vi "Giao tiep 2.vi"() -> ()   [LabVIEW 2020]
uses:
  <vilib>/Instr/_visa.llb/VISA Configure Serial Port (Instr).vi
panel:
  out "concatenated string":string
  in  "BnhanMT":i32(slide) scale=0.0..255.0
  in  "AnhanMT":i32(slide) scale=0.0..255.0
  out "BguiMT":i32
  out "AguiMT":i32
  out "htB":i32(knob) scale=0.0..1000.0
  out "htA":i32(knob) scale=0.0..1023.0
  in  "VISA resource name":refnum<visa-resource-name>="COM10"
  in  "stop":bool
  # "Toc do: 115200"
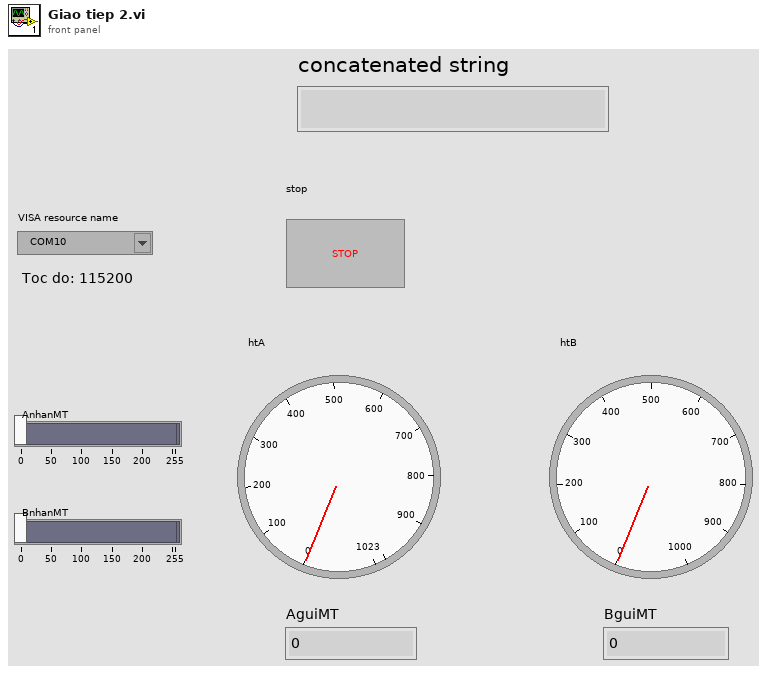
[diagram p1: front panel]
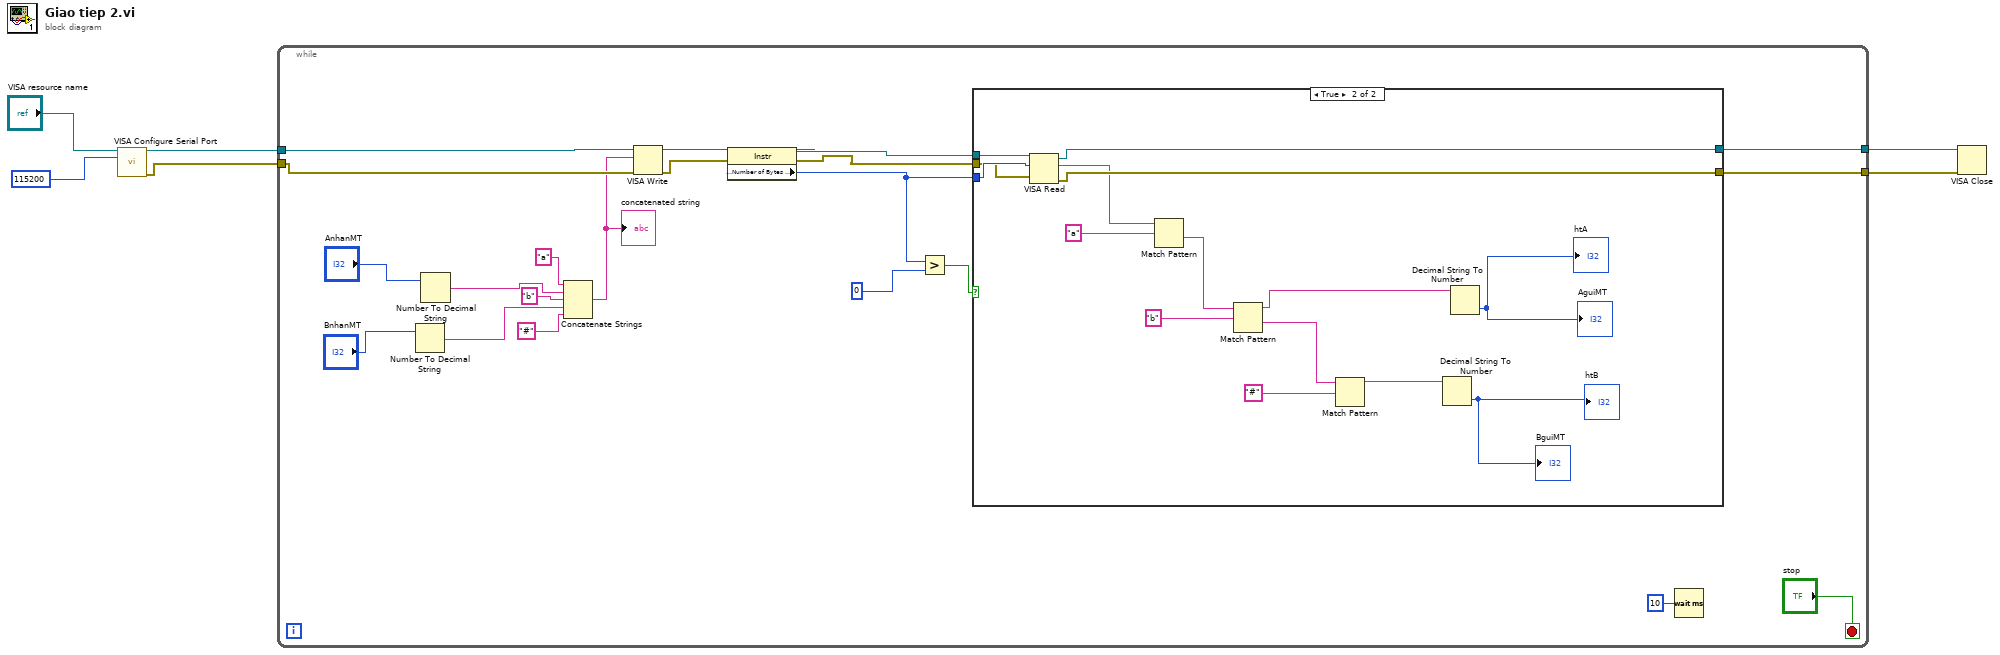
[diagram p0: block diagram]
diagram:
  n1 = call-poly "VISA Configure Serial Port"("VISA resource name"="VISA resource name", "baud rate (9600)"=u32 115200) -> ("VISA resource name out"=w4:refnum<visa-resource-name>, "error out"=w2:errorcluster)  [unwired: 12 in]
  n2 = while {
    tunnel: w4 -> [w21]
    tunnel: [w24] -> w3
    tunnel: w2 -> [w19]
    tunnel: [w22] -> w1
    stop <- "stop" stop-if-true
    n3 = Number To Decimal String(number="BnhanMT") -> (decimal integer string=w9:string)  [unwired: 1 in]
    n4 = Number To Decimal String(number="AnhanMT") -> (decimal integer string=w11:string)  [unwired: 1 in]
    n5 = Concatenate Strings("a" ("string"), w11, "b" ("string"), w9, "#" ("string")) -> (w7:string)
    "concatenated string" <- w7
    n6 = VISA Write(VISA resource name=w21, write buffer=w7, error in (no error)=w19) -> (VISA resource name out=w20:refnum<visa-resource-name>, error out=w18:errorcluster)  [unwired: 1 out]
    n7 = property class="Instr"(reference=w20, error in=w18) -> (reference out=w25:refnum<visa-resource-name>, error out=w23:errorcluster, "Serial Settings:Number of Bytes at Serial Port"=w17:u32)
    n8 = Greater?(x=w17, y=u32 0) -> (0:w15:bool)
    n9 = case shown="True" w15 {
      tunnel: w17 -> [_ w44]
      tunnel: w25 -> [w29 w43]
      tunnel: [w29 w42] -> w24
      tunnel: w23 -> [w28 w41]
      tunnel: [w28 w40] -> w22
      frame False {
      }
      frame True {
        n10 = VISA Read(VISA resource name=w43, byte count=w44, error in (no error)=w41) -> (VISA resource name out=w42:refnum<visa-resource-name>, read buffer=w39:string, error out=w40:errorcluster)  [unwired: 1 out]
        n11 = Match Pattern(string=w39, regular expression="a") -> (after substring=w36:string)  [unwired: 1 in, 3 out]
        n12 = Match Pattern(string=w36, regular expression="b") -> (before substring=w33:string, after substring=w34:string)  [unwired: 1 in, 2 out]
        n13 = Match Pattern(string=w34, regular expression="#") -> (before substring=w31:string)  [unwired: 1 in, 3 out]
        n14 = Decimal String To Number(string=w31) -> (number=→"htB" →"BguiMT":i32)  [unwired: 2 in, 1 out]
        n15 = Decimal String To Number(string=w33) -> (number=→"htA" →"AguiMT":i32)  [unwired: 2 in, 1 out]
      }
    }
    n16 = Wait (ms)(milliseconds to wait=u32 10) -> ()  [unwired: 1 out]
  }
  n17 = VISA Close(VISA resource name=w3, error in (no error)=w1) -> ()  [unwired: 1 out]
